vi "LinxSpiConfigure.vi"(8 "Error In":errorcluster, 9 "SPI Configuration":T1={"Clock Frequency"=1000000, "Bit Order"=enum."LSb First", "SPI Mode"=enum."Mode 0"}, 10 "SPI Channel":u8, 11 "LINX Resource":T4) -> (0 "Error Out":errorcluster, 2 "actualSpeed":u32, 3 "LINX Resource":T4)   [LabVIEW 2014, in "LMH-LINX.lvlib" / "Local IO.lvlib"]
uses:
  <vilib>/MakerHub/LINX/Private/Local IO/Local IO.lvlib
  <vilib>/MakerHub/LINX/Private/Type Defs/LINX Ref.ctl
  <vilib>/MakerHub/LINX/Private/Type Defs/Platform.ctl
  <vilib>/MakerHub/LINX/Private/Type Defs/Interface.ctl
  <vilib>/MakerHub/LINX/Private/Device/Type Defs/LINX Device Config.ctl
  <vilib>/MakerHub/LINX/Private/Device/Type Defs/TCP Config.ctl
  <vilib>/MakerHub/LINX/Private/Device/Type Defs/Channels.ctl
  <vilib>/MakerHub/LINX/Private/Type Defs/Peripherals/SPI/SPI Configuration.ctl
  <vilib>/MakerHub/LINX/Private/Type Defs/Peripherals/SPI/SPI Bit Order.ctl
  <vilib>/MakerHub/LINX/Private/Type Defs/Peripherals/SPI/SPI Mode.ctl
  <vilib>/MakerHub/LINX/Private/Type Defs/Error Type.ctl
  <vilib>/MakerHub/LINX/LMH-LINX.lvlib
  <vilib>/MakerHub/LINX/Private/Type Defs/Channel FGV States.ctl
  <vilib>/myRIO/Common/Instrument Driver Framework/myRIO v1.0/SPI/typedefs/SPI Frame Length.ctl
  <vilib>/myRIO/Common/Instrument Driver Framework/myRIO v1.0/SPI/typedefs/SPI Data Direction.ctl
  <vilib>/myRIO/Common/Instrument Driver Framework/myRIO v1.0/SPI/typedefs/SPI Clock Polarity.ctl
  <vilib>/myRIO/Common/Instrument Driver Framework/myRIO v1.0/SPI/typedefs/SPI Clock Phase.ctl
  <vilib>/myRIO/Instrument Drivers/Onboard IO/SPI/typedefs/SPI Configuration.ctl
  <vilib>/myRIO/Common/Instrument Driver Framework/myRIO v1.0/SPI/typedefs/SPI Channels Enum.ctl
  <vilib>/myRIO/Common/Instrument Driver Framework/Utilities/typedefs/Generic FPGA Reference.ctl
  <vilib>/myRIO/Common/Instrument Driver Framework/Utilities/typedefs/myRIO v1.0 Reference.ctl
  <vilib>/myRIO/Common/Instrument Driver Framework/Utilities/typedefs/Hardware Version Enum.ctl
  <vilib>/myRIO/Common/Instrument Driver Framework/Utilities/typedefs/myRIO Generic Hardware Reference.ctl
  <vilib>/myRIO/Instrument Drivers/Onboard IO/SPI/typedefs/SPI Reference.ctl
  <vilib>/myRIO/Instrument Drivers/Onboard IO/SPI/SPI.lvlib
  liblinxdevice.dll
  <vilib>/MakerHub/LINX/Private/Device/Device.lvlib
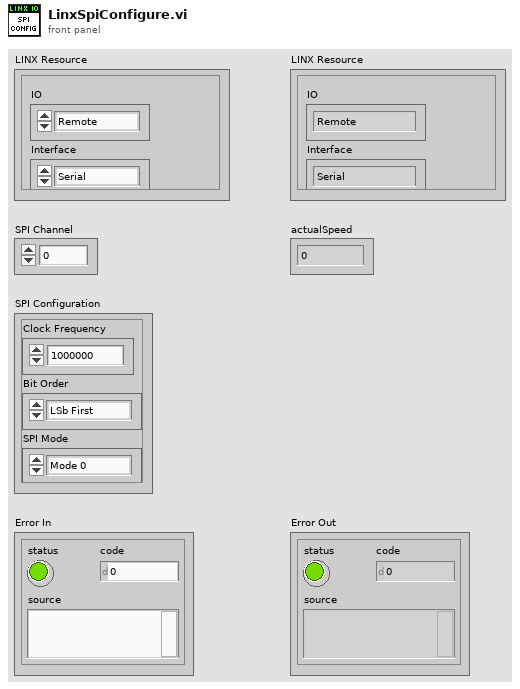
[diagram p1: front panel]
types:
  T1 = typedef "LMH-LINX.lvlib/SPI Configuration.ctl" = cluster{"Clock Frequency":u32, "Bit Order":T2, "SPI Mode":T3}
  T2 = typedef "LMH-LINX.lvlib/SPI Bit Order.ctl" = enum8{"LSb First", "MSb First"}
  T3 = typedef "LMH-LINX.lvlib/SPI Mode.ctl" = enum8{"Mode 0", "Mode 1", "Mode 2", "Mode 3"}
  T4 = typedef "LMH-LINX.lvlib/LINX Ref.ctl" = cluster{"IO":T5, "Interface":T6, "LINX Device Config":T7}
  T5 = typedef "LMH-LINX.lvlib/Platform.ctl" = enum16{"Remote", "Local"}
  T6 = typedef "LMH-LINX.lvlib/Interface.ctl" = enum16{"Serial", "TCP"}
  T7 = typedef "LMH-LINX.lvlib/Device.lvlib/LINX Device Config.ctl" = cluster{"Interface":T6, "COM Port":refnum<visa-resource-name>, "TCP Configuration":T8, "Device Family":u8, "Device ID":u8, "Device Name":string, "TCP Ref":refnum<k5>, "Channels":T9}
  T8 = typedef "LMH-LINX.lvlib/Device.lvlib/TCP Config.ctl" = cluster{"IP Address":string, "Port":u16}
  T9 = typedef "LMH-LINX.lvlib/Channels.ctl" = cluster{"DI":u8[], "DO":u8[], "AI":u8[], "AO":u8[], "PWM":u8[], "QE":u8[], "UART":u8[], "I2C 2":u8[], "SPI":u8[], "CAN":u8[], "Servo":u8[], "AI Ref (V)":dbl, "AI Resolution (Bits)":u8, "AO Ref (V)":dbl, "AO Resolution (Bits)":u8}
  T10 = typedef "LMH-LINX.lvlib/Error Type.ctl" = enum16{"Unknown", "Timeout", "Corrupt Return Packet", "Unable To Connect", "Command Not Supported", "Channel DNE", "Invalid COM Config", "Firmware Version Mismatch", "myRIO Support", "CMD Specific Error", "Local IO Not Supported"}
  T11 = cluster{"Frequency":dbl, "Clock Phase":u8, "Clock Polarity":u8, "Data Direction":u8, "Frame Length":u8}
  T12 = typedef "LMH-LINX.lvlib/Channel FGV States.ctl" = enum16{"Initialize", "Get", "Set"}
  T13 = typedef "SPI.lvlib/SPI Reference.ctl" = cluster{"myRIO Reference":T14, "SPI Channels Enum":T18, "SPI Configuration":T19}
  T14 = typedef "myRIO Generic Hardware Reference.ctl" = cluster{"myRIO Model":T15, "myRIO Hardware Reference":T16}
  T15 = typedef "Hardware Version Enum.ctl" = enum16{"Unknown", "myRIO-1900", "myRIO-1950"}
  T16 = typedef "myRIO v1.0 Reference.ctl" = cluster{"Generic FPGA Reference":T17, "Allow multiple opens":bool}
  T17 = typedef "Generic FPGA Reference.ctl" = refnum<k20>
  T18 = typedef "SPI Channels Enum.ctl" = enum16{"Not Connected", "A/SPI", "B/SPI"}
  T19 = typedef "SPI.lvlib/SPI Configuration.ctl" = cluster{"Frequency [Hz]":dbl, "Clock Phase":T20, "Clock Polarity":T21, "Data Direction":T22, "Frame Length":T23}
  T20 = typedef "SPI Clock Phase.ctl" = enum8{"Leading", "Trailing"}
  T21 = typedef "SPI Clock Polarity.ctl" = enum8{"Low", "High"}
  T22 = typedef "SPI Data Direction.ctl" = enum8{"Most significant bit first", "Least significant bit first"}
  T23 = typedef "SPI Frame Length.ctl" = u8
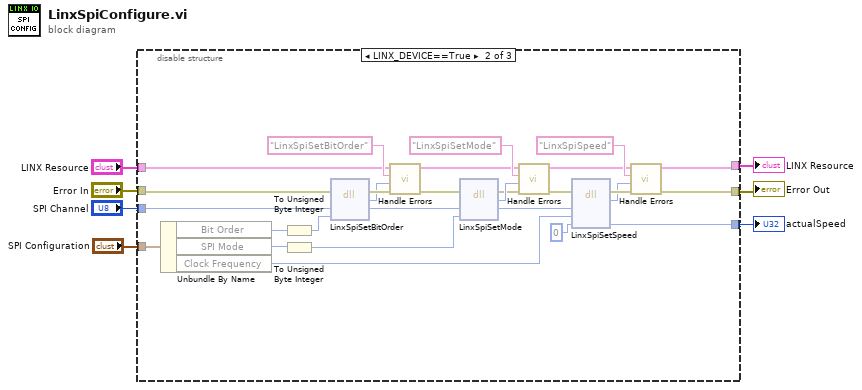
[diagram p0: block diagram]
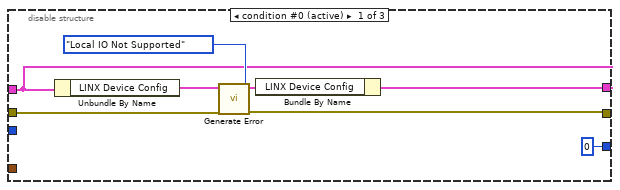
[diagram p2: hidden frame]
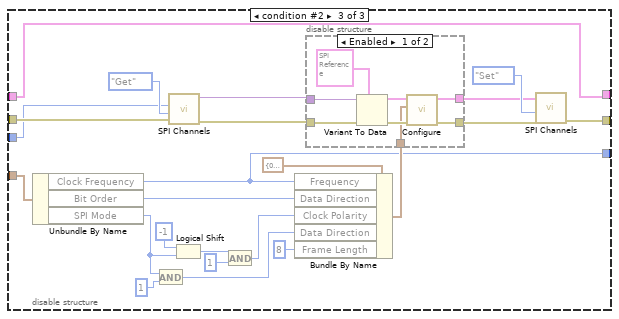
[diagram p3: hidden frame]
diagram:
  n1 = disable-structure shown="LINX_DEVICE==True" {
    disable-tunnel: [w10 w17 w45] -> w7
    disable-tunnel: "LINX Resource" -> [w12 w38 w45]
    disable-tunnel: "Error In" -> [w14 w41 w50]
    disable-tunnel: "SPI Channel" -> [_ w39 w48]
    disable-tunnel: "SPI Configuration" -> [_ w37 w49]
    disable-tunnel: [u32 0 ("actualSpeed") w18 w46] -> w2
    disable-tunnel: [w8 w16 w44] -> w1
    frame condition #0 (active) {
      n2 = Unbundle By Name(w12) -> ("LINX Device Config"=w13:T7)
      n3 = call <vilib>:"Generate Error.vi"("Error In"=w14, "Error Type"=Error_Type."Local IO Not Supported", "LINX Device Config"=w13) -> ("Error Out"=w8:errorcluster, "Dup LINX Device Config"=w11:T7)  [unwired: 7 in]
      n4 = Bundle By Name(cluster=w12, "LINX Device Config"=w11) -> (w10:T4)
    }
    frame condition #1 {
      n5 = Unbundle By Name(w37) -> ("Bit Order"=w36:T2, "SPI Mode"=w28:T3, "Clock Frequency"=w20:u32)
      n6 = To Unsigned Byte Integer(number=w36) -> (unsigned 8bit integer=w35:u8)
      n7 = To Unsigned Byte Integer(number=w28) -> (unsigned 8bit integer=w27:u8)
      n8 = dll-call lib="liblinxdevice.*" fn="LinxSpiSetBitOrder"(error in=w41, "channel"=w39, "bitOrder"=w35) -> (error out=w42:errorcluster, "Status"=w40:i32, "channel"=w29:u8)  [unwired: 3 in, 1 out]
      n9 = call <vilib>:"Handle Errors.vi"("Error In"=w42, "LinxStatus"=w40, "Function Name"="LinxSpiSetBitOrder", "LINX Resource"=w38) -> ("Error Out"=w31:errorcluster, "LINX Resource"=w30:T4)  [unwired: 6 in]
      n10 = dll-call lib="liblinxdevice.*" fn="LinxSpiSetMode"(error in=w31, "channel"=w29, "mode"=w27) -> (error out=w33:errorcluster, "Status"=w34:i32, "channel"=w21:u8)  [unwired: 3 in, 1 out]
      n11 = call <vilib>:"Handle Errors.vi"("Error In"=w33, "LinxStatus"=w34, "Function Name"="LinxSpiSetMode", "LINX Resource"=w30) -> ("Error Out"=w23:errorcluster, "LINX Resource"=w22:T4)  [unwired: 6 in]
      n12 = dll-call lib="liblinxdevice.*" fn="LinxSpiSetSpeed"(error in=w23, "channel"=w21, "speed"=w20, "actualSpeed"=u32 0) -> (error out=w25:errorcluster, "Status"=w24:i32, "actualSpeed"=w18:u32)  [unwired: 4 in, 1 out]
      n13 = call <vilib>:"Handle Errors.vi"("Error In"=w25, "LinxStatus"=w24, "Function Name"="LinxSpiSpeed", "LINX Resource"=w22) -> ("Error Out"=w16:errorcluster, "LINX Resource"=w17:T4)  [unwired: 6 in]
    }
    frame condition #2 {
      n14 = Unbundle By Name(w49) -> ("Clock Frequency"=w46:u32, "Bit Order"=w57:T2, "SPI Mode"=w55:T3)
      n15 = And(x=w55, y=u8 1 ("Frame Length")) -> (x .and. y?=w56:u8)
      n16 = call <vilib>:"SPI Channels.vi"("Error In"=w50, "Channel State"=Channel_FGV_States."Get", "Channel Number"=w48) -> ("Error Out"=w64:errorcluster, "SPI Channel"=w59:variant)  [unwired: 7 in]
      n17 = Logical Shift(y=i8 -1, x=w55) -> (x << y=w52:u32)
      n18 = And(x=w52, y=u8 1 ("Frame Length")) -> (x .and. y?=w51:u32)
      n19 = Bundle By Name(cluster=T11 {"Frequency"=0.0, "Clock Phase"=0, "Clock Polarity"=0, "Data Direction"=0, "Frame Length"=0}, "Frequency"=w46, "Data Direction"=w57, "Clock Polarity"=w51, "Data Direction"=w56, "Frame Length"=u8 8) -> (w58:T11)
      n20 = disable-structure shown="Enabled" {
        disable-tunnel: w64 -> [w71 _]
        disable-tunnel: [w70 _] -> w63
        disable-tunnel: [w69 _] -> w60
        disable-tunnel: w59 -> [w68 _]
        disable-tunnel: w58 -> [w67 _]
        frame Enabled {
          n21 = Variant To Data(error in=w71, type=T13 {"myRIO Reference"={"myRIO Model"=enum."Unknown", "myRIO Hardware Reference"={"Generic FPGA Reference"=refnum, "Allow multiple opens"=FALSE}}, "SPI Channels Enum"=enum."Not Connected", "SPI Configuration"={"Frequency [Hz]"=0.0, "Clock Phase"=enum."Leading", "Clock Polarity"=enum."Low", "Data Direction"=enum."Most significant bit first", "Frame Length"=8}} ("SPI Ref In"), Variant=w68) -> (data=w73:T13, error out=w72:errorcluster)
          n22 = call <vilib>:"Configure.vi"("error in (no error)"=w72, "SPI User Configuration"=w67, "SPI Ref In"=w73) -> ("error out"=w70:errorcluster, "SPI Ref Out"=w69:T13)  [unwired: 7 in]
        }
        frame Disabled {
        }
      }
      n23 = call <vilib>:"SPI Channels.vi"("Error In"=w63, "Channel State"=Channel_FGV_States."Set", "SPI Channel"=w60) -> ("Error Out"=w44:errorcluster)  [unwired: 7 in, 1 out]
    }
  }
  "LINX Resource" <- w7
  "Error Out" <- w1
  "actualSpeed" <- w2
